vi "GetDataEventProperties.vi"(9 "data":T4, 10 "device name":string, 11 "data event config":T1) -> (2 "data event properties":T7[](array[typedef]))   [LabVIEW 2017, in "EmsaDataEventCreator.lvlib"]
uses:
  <vilib>/addons/InsightCM/Devices/Shared/Emsa/EmsaDataEventCreator/EmsaDataEventCreator.lvlib
  <vilib>/addons/InsightCM/MessageBus/Base/controls/KeyValuePair.ctl
  <vilib>/addons/InsightCM/Devices/Shared/Common/DataFlow/controls/Data.ctl
  <vilib>/addons/InsightCM/Utilities/DataAccessors/controls/wfmSGL_DVR.ctl
  <vilib>/addons/PointValueMap/controls/PointMap.ctl
  <vilib>/addons/InsightCM/Devices/Shared/Common/DataFlow/controls/Type.ctl
  <vilib>/addons/InsightCM/Devices/Shared/Emsa/EmsaDataEventCreator/controls/DataEventConfig.ctl
  <vilib>/addons/InsightCM/Devices/Shared/Emsa/EmsaDataEventCreator/controls/SweepParams.ctl
  <vilib>/addons/InsightCM/Utilities/PropertyHelpers/PropertyHelpers.lvlib
  <vilib>/addons/InsightCM/Devices/Shared/Common/DataFlow/DataFlow.lvlib
  <vilib>/addons/PointValueMap/PointValueMap.lvlib
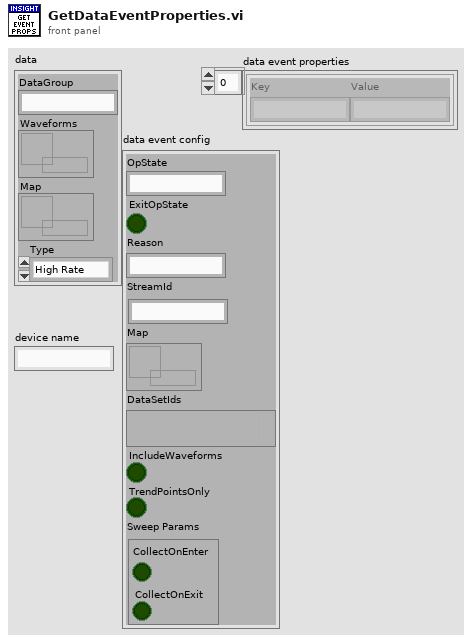
[diagram p1: front panel]
types:
  T1 = typedef "EmsaDataEventCreator.lvlib/DataEventConfig.ctl" = cluster{"OpState":string, "ExitOpState":bool, "Reason":string, "StreamId":string, "Map":T2, "DataSetIds":variant, "IncludeWaveforms":bool, "TrendPointsOnly":bool, "Sweep Params":T3}
  T2 = typedef "PointValueMap.lvlib/PointMap.ctl" = refnum<data-value>
  T3 = typedef "EmsaDataEventCreator.lvlib/SweepParams.ctl" = cluster{"CollectOnEnter":bool, "CollectOnExit":bool}
  T4 = typedef "DataFlow.lvlib/Data.ctl" = cluster{"DataGroup":string, "Waveforms":T5, "Map":T2, "Type":T6}
  T5 = typedef "wfmSGL_DVR.ctl" = refnum<data-value>
  T6 = typedef "DataFlow.lvlib/Type.ctl" = enum16{"High Rate", "Low Rate", "Burst Mode"}
  T7 = typedef "KeyValuePair.ctl" = cluster{"Key":string, "Value":string}
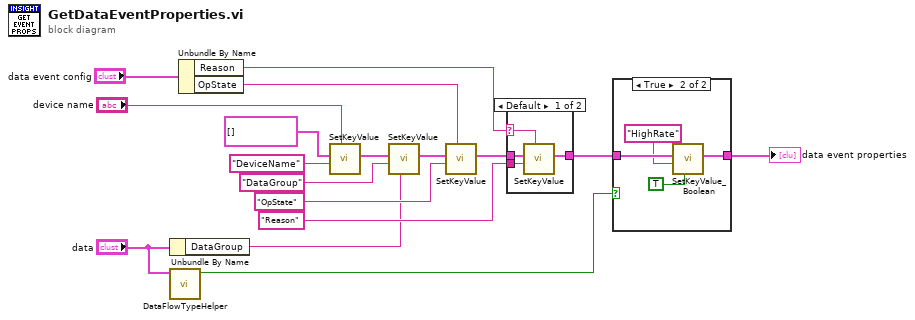
[diagram p0: block diagram]
diagram:
  n1 = Unbundle By Name("data") -> ("DataGroup"=w6:string)
  n2 = call <vilib>:"DataFlowTypeHelper.vi"("data"="data") -> ("high rate"=w1:bool)  [unwired: 8 in, 2 out]
  n3 = Unbundle By Name("data event config") -> ("Reason"=w17:string, "OpState"=w16:string)
  n4 = call <vilib>:"SetKeyValue.vi"("value"="device name", "key"="DeviceName", "key value pairs"=T7[] []) -> ("key value pairs out"=w9:T7[])  [unwired: 8 in]
  n5 = call <vilib>:"SetKeyValue.vi"("value"=w6, "key"="DataGroup", "key value pairs"=w9) -> ("key value pairs out"=w10:T7[])  [unwired: 8 in]
  n6 = call <vilib>:"SetKeyValue.vi"("value"=w16, "key"="OpState", "key value pairs"=w10) -> ("key value pairs out"=w13:T7[])  [unwired: 8 in]
  n7 = case shown="Default" w17 {
    selector: w17 -> [w18 _]
    tunnel: w13 -> [w21 w22]
    tunnel: "Reason" ("key") -> [w20 _]
    tunnel: [w19 w22] -> w3
    frame Default {
      n8 = call <vilib>:"SetKeyValue.vi"("value"=w18, "key"=w20, "key value pairs"=w21) -> ("key value pairs out"=w19:T7[])  [unwired: 8 in]
    }
    frame "" {
    }
  }
  n9 = case shown="True" w1 {
    tunnel: [w23 w26] -> w5
    tunnel: w3 -> [w23 w27]
    frame False {
    }
    frame True {
      n10 = call <vilib>:"SetKeyValue_Boolean.vi"("value"=TRUE, "key"="HighRate", "key value pairs"=w27) -> ("key value pairs out"=w26:T7[])  [unwired: 8 in]
    }
  }
  "data event properties" <- w5
